vi "BBoxLite28A.vi"() -> ()   [LabVIEW 2020]
uses:
  Y:/Documents/TMYtek/Code/bbox-api/example/BBoxLite Series/LabVIEW/BBoxLite28A/BBoxAPI.dll
  BBoxAPI.dll
panel:
  out "setBeamAngle":i32(ring)=13 items=["OK"=0, "WARNING"=1, "ERROR"=2, "NO_RESPONSE"=3, "ERROR_GET_SN"=10, "ERROR_DEV_TYPE"=11, "ERROR_INIT_OBJECT"=12, "ERROR_DEV_NOT_INIT"=13, "ERROR_METHOD_NOT_FOUND"=14, "ERROR_REFLECTION"=15, "ERROR_POWER"=16, "ERROR_NETWORK_NOT_INIT"=20, "ERROR_NETWORK_INIT"=21, "ERROR_NETWORK_CONNECT_TIMEOUT"=22, "ERROR_DISCONNECT"=23, "ERROR_SOCKET"=24, "ERROR_SEND_CMD"=25, "ERROR_RESP_CMD"=26, "ERROR_DEV_COUNT_ZERO"=30, "ERROR_CMD"=40, "ERROR_CMD_INIT"=41, "ERROR_BF_AAKIT"=100, "ERROR_BF_NO_AAKIT"=101, "ERROR_BF_CALI_PATH"=102, "ERROR_BF_BEAMXY"=103, "ERROR_BF_GEN"=104, "ERROR_BF_TRMODE"=105, "STATUS_BF_LOAD_CALI_INCOMPLTE"=106, "ERROR_BF_LOAD_CALI_PARSE_FAILED"=107, "ERROR_FREQ_EQUATION"=250, "ERROR_PLO_CRC"=251, "WARNING_HARMONIC"=252, "ERROR_HARMONIC_BLOCK"=253]
  in  "Your AAKit Name":string="TMYTEK_28LITE_4x4_C2104L020-28"
  out "getAAKitList":string[](array[string])
  in  "Phi":i32 min=-45 max=45 step=1
  out "switchChannelPower":string
  in  "Power":i32
  out "selectAAKit":i32(ring)=13 items=["OK"=0, "WARNING"=1, "ERROR"=2, "NO_RESPONSE"=3, "ERROR_GET_SN"=10, "ERROR_DEV_TYPE"=11, "ERROR_INIT_OBJECT"=12, "ERROR_DEV_NOT_INIT"=13, "ERROR_METHOD_NOT_FOUND"=14, "ERROR_REFLECTION"=15, "ERROR_POWER"=16, "ERROR_NETWORK_NOT_INIT"=20, "ERROR_NETWORK_INIT"=21, "ERROR_NETWORK_CONNECT_TIMEOUT"=22, "ERROR_DISCONNECT"=23, "ERROR_SOCKET"=24, "ERROR_SEND_CMD"=25, "ERROR_RESP_CMD"=26, "ERROR_DEV_COUNT_ZERO"=30, "ERROR_CMD"=40, "ERROR_CMD_INIT"=41, "ERROR_BF_AAKIT"=100, "ERROR_BF_NO_AAKIT"=101, "ERROR_BF_CALI_PATH"=102, "ERROR_BF_BEAMXY"=103, "ERROR_BF_GEN"=104, "ERROR_BF_TRMODE"=105, "STATUS_BF_LOAD_CALI_INCOMPLTE"=106, "ERROR_BF_LOAD_CALI_PARSE_FAILED"=107, "ERROR_FREQ_EQUATION"=250, "ERROR_PLO_CRC"=251, "WARNING_HARMONIC"=252, "ERROR_HARMONIC_BLOCK"=253]
  out "readBeamPhaseValues":i32[][](array[numeric])
  out "readBeamGainValues":dbl[][](array[numeric])
  in  "Theta":i32 min=-45 max=45 step=1
  in  "Beam Gain":dbl step=0.5
  out "setChannelGainPhase":string
  in  "Phase":i32 min=0 max=355 step=5
  in  "Gain":dbl=18.0 step=0.5
  in  "Channel":i32=1 min=1 max=4
  in  "TxRxMode":i32=1 min=1 max=2 step=1
  out "Maxmum Gain":dbl
  out "Minimum Gain":dbl
  out "getTxRxMode":i32
  out "SwitchTxRxMode":i32(ring) items=["OK"=0, "WARNING"=1, "ERROR"=2, "NO_RESPONSE"=3, "ERROR_GET_SN"=10, "ERROR_DEV_TYPE"=11, "ERROR_INIT_OBJECT"=12, "ERROR_DEV_NOT_INIT"=13, "ERROR_METHOD_NOT_FOUND"=14, "ERROR_REFLECTION"=15, "ERROR_POWER"=16, "ERROR_NETWORK_NOT_INIT"=20, "ERROR_NETWORK_INIT"=21, "ERROR_NETWORK_CONNECT_TIMEOUT"=22, "ERROR_DISCONNECT"=23, "ERROR_SOCKET"=24, "ERROR_SEND_CMD"=25, "ERROR_RESP_CMD"=26, "ERROR_DEV_COUNT_ZERO"=30, "ERROR_CMD"=40, "ERROR_CMD_INIT"=41, "ERROR_BF_AAKIT"=100, "ERROR_BF_NO_AAKIT"=101, "ERROR_BF_CALI_PATH"=102, "ERROR_BF_BEAMXY"=103, "ERROR_BF_GEN"=104, "ERROR_BF_TRMODE"=105, "STATUS_BF_LOAD_CALI_INCOMPLTE"=106, "ERROR_BF_LOAD_CALI_PARSE_FAILED"=107, "ERROR_FREQ_EQUATION"=250, "ERROR_PLO_CRC"=251, "WARNING_HARMONIC"=252, "ERROR_HARMONIC_BLOCK"=253]
  out "setOperatingFreq":i32(ring)=13 items=["OK"=0, "WARNING"=1, "ERROR"=2, "NO_RESPONSE"=3, "ERROR_GET_SN"=10, "ERROR_DEV_TYPE"=11, "ERROR_INIT_OBJECT"=12, "ERROR_DEV_NOT_INIT"=13, "ERROR_METHOD_NOT_FOUND"=14, "ERROR_REFLECTION"=15, "ERROR_POWER"=16, "ERROR_NETWORK_NOT_INIT"=20, "ERROR_NETWORK_INIT"=21, "ERROR_NETWORK_CONNECT_TIMEOUT"=22, "ERROR_DISCONNECT"=23, "ERROR_SOCKET"=24, "ERROR_SEND_CMD"=25, "ERROR_RESP_CMD"=26, "ERROR_DEV_COUNT_ZERO"=30, "ERROR_CMD"=40, "ERROR_CMD_INIT"=41, "ERROR_BF_AAKIT"=100, "ERROR_BF_NO_AAKIT"=101, "ERROR_BF_CALI_PATH"=102, "ERROR_BF_BEAMXY"=103, "ERROR_BF_GEN"=104, "ERROR_BF_TRMODE"=105, "STATUS_BF_LOAD_CALI_INCOMPLTE"=106, "ERROR_BF_LOAD_CALI_PARSE_FAILED"=107, "ERROR_FREQ_EQUATION"=250, "ERROR_PLO_CRC"=251, "WARNING_HARMONIC"=252, "ERROR_HARMONIC_BLOCK"=253]
  out "getFrequencyList":string[](array[string])
  out "Init":i32(ring)=13 items=["OK"=0, "WARNING"=1, "ERROR"=2, "NO_RESPONSE"=3, "ERROR_GET_SN"=10, "ERROR_DEV_TYPE"=11, "ERROR_INIT_OBJECT"=12, "ERROR_DEV_NOT_INIT"=13, "ERROR_METHOD_NOT_FOUND"=14, "ERROR_REFLECTION"=15, "ERROR_POWER"=16, "ERROR_NETWORK_NOT_INIT"=20, "ERROR_NETWORK_INIT"=21, "ERROR_NETWORK_CONNECT_TIMEOUT"=22, "ERROR_DISCONNECT"=23, "ERROR_SOCKET"=24, "ERROR_SEND_CMD"=25, "ERROR_RESP_CMD"=26, "ERROR_DEV_COUNT_ZERO"=30, "ERROR_CMD"=40, "ERROR_CMD_INIT"=41, "ERROR_BF_AAKIT"=100, "ERROR_BF_NO_AAKIT"=101, "ERROR_BF_CALI_PATH"=102, "ERROR_BF_BEAMXY"=103, "ERROR_BF_GEN"=104, "ERROR_BF_TRMODE"=105, "STATUS_BF_LOAD_CALI_INCOMPLTE"=106, "ERROR_BF_LOAD_CALI_PARSE_FAILED"=107, "ERROR_FREQ_EQUATION"=250, "ERROR_PLO_CRC"=251, "WARNING_HARMONIC"=252, "ERROR_HARMONIC_BLOCK"=253]
  out "SN":string
  out "ScanningDevice":string[](array[string])
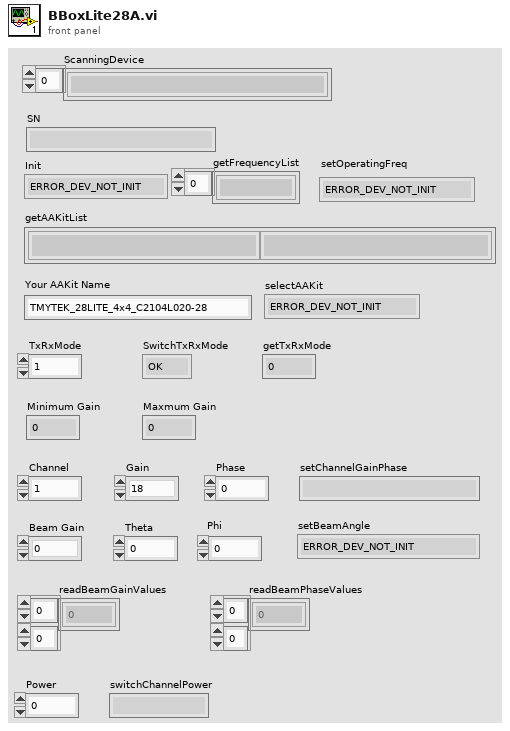
[diagram p1: front panel]
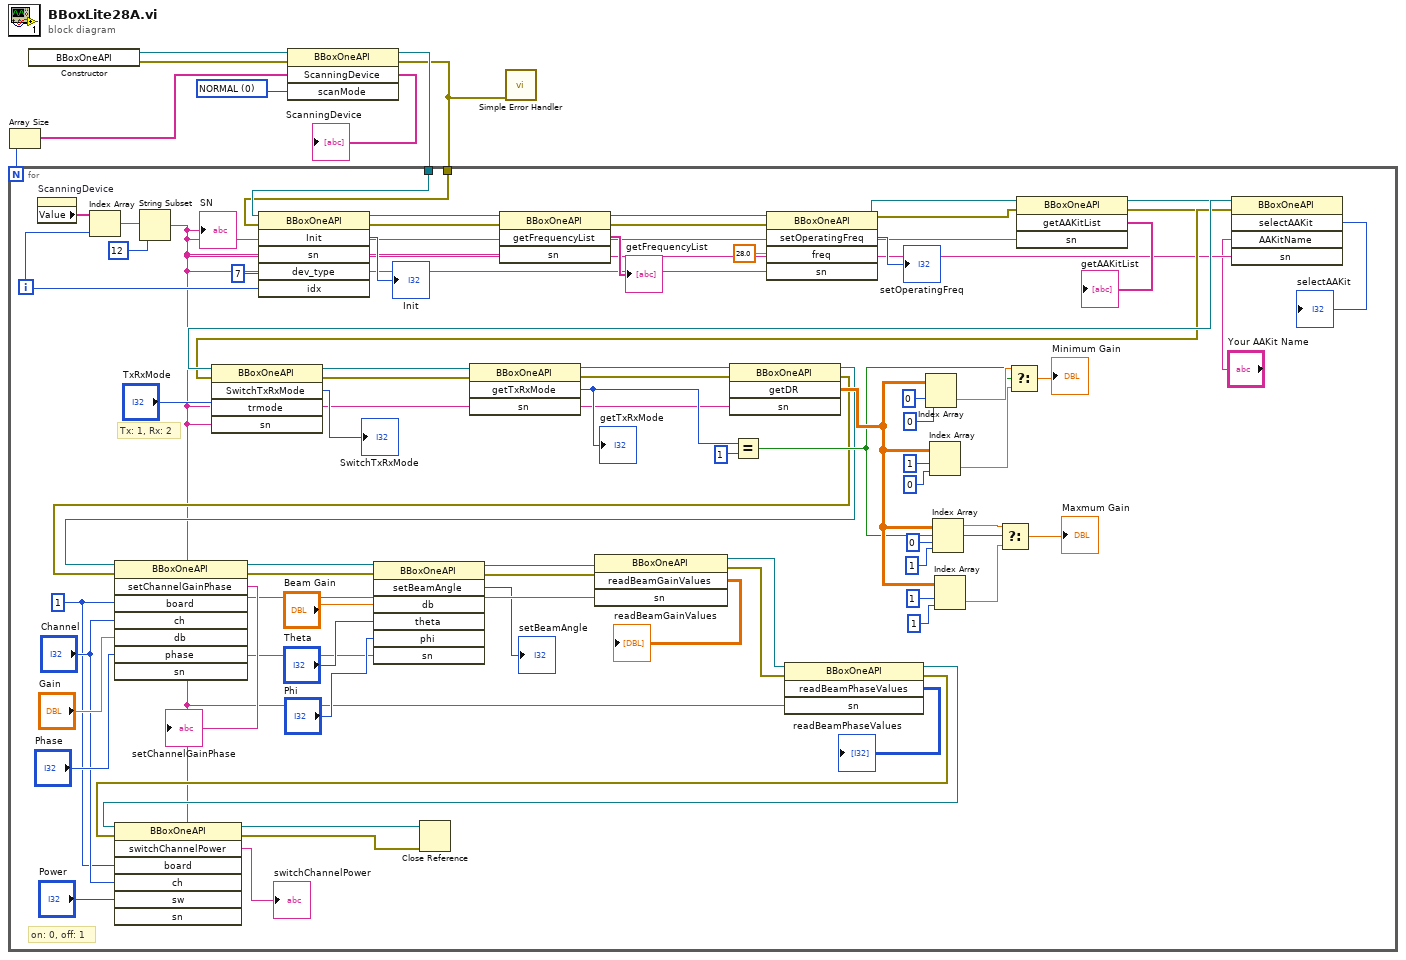
[diagram p0: block diagram]
diagram:
  w7 = 0 items=["NORMAL", "FAST"] ("scanMode")
  n1 = constructor class="BBoxOneAPI"() -> (reference out=w6:refnum<k24>, error out=w5:errorcluster)  [unwired: 3 in, 1 out]
  n2 = invoke class="BBoxOneAPI" method="ScanningDevice"(reference=w6, error in=w5, "scanMode"=w7) -> (reference out=w2:refnum<k24>, error out=w1:errorcluster, "ScanningDevice"=w3:string[])  [unwired: 1 in, 1 out]
  "ScanningDevice" <- w3
  n3 = Array Size(array=w3) -> (size(s)=w4:i32)
  n4 = for {
    N: w4 -> [_]
    tunnel: w2 -> [w79]
    tunnel: w1 -> [w78]
    i -> [w76]
    w27 = 1
    # "on: 0, off: 1"
    # "Tx: 1, Rx: 2"
    n5 = property on="ScanningDevice" class="Arr (strict)"() -> ("Value"=w18:string[])  [unwired: 2 in, 2 out]
    n6 = Index Array(array=w18, index=w76) -> (element=w81:string)
    n7 = String Subset(string=w81, length (rest)=12) -> (substring=w12:string)  [unwired: 1 in]
    "SN" <- w12
    n8 = invoke class="BBoxOneAPI" method="Init"(reference=w79, error in=w78, "sn"=w12, "dev_type"=7, "idx"=w76) -> (reference out=w17:refnum<k24>, error out=w16:errorcluster, "Init"=→"Init":i32)  [unwired: 1 in, 3 out]
    n9 = invoke class="BBoxOneAPI" method="getFrequencyList"(reference=w17, error in=w16, "sn"=w12) -> (reference out=w15:refnum<k24>, error out=w14:errorcluster, "getFrequencyList"=→"getFrequencyList":string[])  [unwired: 1 in, 1 out]
    n10 = invoke class="BBoxOneAPI" method="setOperatingFreq"(reference=w15, error in=w14, "freq"=28.0, "sn"=w12) -> (reference out=w23:refnum<k24>, error out=w22:errorcluster, "setOperatingFreq"=→"setOperatingFreq":i32)  [unwired: 1 in, 2 out]
    n11 = invoke class="BBoxOneAPI" method="getAAKitList"(reference=w23, error in=w22, "sn"=w12) -> (reference out=w21:refnum<k24>, error out=w20:errorcluster, "getAAKitList"=→"getAAKitList":string[])  [unwired: 1 in, 1 out]
    n12 = invoke class="BBoxOneAPI" method="selectAAKit"(reference=w21, error in=w20, "AAKitName"="Your AAKit Name", "sn"=w12) -> (reference out=w33:refnum<k24>, error out=w32:errorcluster, "selectAAKit"=→"selectAAKit":i32)  [unwired: 1 in, 2 out]
    n13 = invoke class="BBoxOneAPI" method="SwitchTxRxMode"(reference=w33, error in=w32, "trmode"="TxRxMode", "sn"=w12) -> (reference out=w71:refnum<k24>, error out=w70:errorcluster, "SwitchTxRxMode"=→"SwitchTxRxMode":i32)  [unwired: 1 in, 2 out]
    n14 = invoke class="BBoxOneAPI" method="getTxRxMode"(reference=w71, error in=w70, "sn"=w12) -> (reference out=w69:refnum<k24>, error out=w68:errorcluster, "getTxRxMode"=w67:i32)  [unwired: 1 in, 1 out]
    "getTxRxMode" <- w67
    n15 = invoke class="BBoxOneAPI" method="getDR"(reference=w69, error in=w68, "sn"=w12) -> (reference out=w48:refnum<k24>, error out=w47:errorcluster, "getDR"=w56:dbl[][])  [unwired: 1 in, 1 out]
    n16 = invoke class="BBoxOneAPI" method="setChannelGainPhase"(reference=w48, error in=w47, "board"=w27, "ch"="Channel", "db"="Gain", "phase"="Phase", "sn"=w12) -> (reference out=w43:refnum<k24>, error out=w42:errorcluster, "setChannelGainPhase"=→"setChannelGainPhase":string)  [unwired: 1 in, 5 out]
    n17 = invoke class="BBoxOneAPI" method="setBeamAngle"(reference=w43, error in=w42, "db"="Beam Gain", "theta"="Theta", "phi"="Phi", "sn"=w12) -> (reference out=w39:refnum<k24>, error out=w38:errorcluster, "setBeamAngle"=→"setBeamAngle":i32)  [unwired: 1 in, 4 out]
    n18 = invoke class="BBoxOneAPI" method="readBeamGainValues"(reference=w39, error in=w38, "sn"=w12) -> (reference out=w36:refnum<k24>, error out=w35:errorcluster, "readBeamGainValues"=→"readBeamGainValues":dbl[][])  [unwired: 1 in, 1 out]
    n19 = Equal?(x=w67, y=1) -> (x = y?=w53:bool)
    n20 = invoke class="BBoxOneAPI" method="readBeamPhaseValues"(reference=w36, error in=w35, "sn"=w12) -> (reference out=w30:refnum<k24>, error out=w29:errorcluster, "readBeamPhaseValues"=→"readBeamPhaseValues":i32[][])  [unwired: 1 in, 1 out]
    n21 = invoke class="BBoxOneAPI" method="switchChannelPower"(reference=w30, error in=w29, "board"=w27, "ch"="Channel", "sw"="Power", "sn"=w12) -> (reference out=w10:refnum<k24>, error out=w11:errorcluster, "switchChannelPower"=→"switchChannelPower":string)  [unwired: 1 in, 4 out]
    n22 = Close Reference(reference=w10, error in (no error)=w11) -> ()  [unwired: 1 out]
    n23 = Index Array(array=w56, index (row)=0, index (col)=0) -> (element=w63:dbl)
    n24 = Index Array(array=w56, index (row)=1, index (col)=0) -> (element=w60:dbl)
    n25 = Index Array(array=w56, index (row)=0, index (col)=1) -> (element=w52:dbl)
    n26 = Index Array(array=w56, index (row)=1, index (col)=1) -> (element=w51:dbl)
    n27 = Select(t=w52, s=w53, f=w51) -> (s? t:f=→"Maxmum Gain":dbl)
    n28 = Select(t=w63, s=w53, f=w60) -> (s? t:f=→"Minimum Gain":dbl)
  }
  n29 = call <vilib>:"Simple Error Handler.vi"("error in (no error)"=w1) -> ()  [unwired: 4 in, 5 out]
